vi "WLAN_DPD_AMPM_EVM_SEM.vi"() -> ()   [LabVIEW 2016]
doc: "This example illustrates how to use the RFmx and RFSG drivers and the WLAN toolkit to perform SEM and EVM measurements with or without digital predistortion (DPD) of the waveform input to the DUT. \n\nDPD is a technique to optimize the operating point of power amplifiers and other non-linear RFIC devices. Power amplifiers are much more efficient if they operate near compression. However, compressing signal amplitudes can significantly deteriorate the amplified signal's quality both, in-band (e.g., EVM increases due to non-linear distortion of the signal's I/Q constellation) and out-of-band (e.g., SEM test fails due to spectral regrowth). With DPD, the original waveform is first pre-distorted in a way that matches the non-linear effects of the RFIC device before being fed through the device. The resulting output is a much cleaner amplified and/or filtered version of the original waveform. \n\nDifferent DPD models can be used to trade off performance with computational ease, with the Lookup-Table (LUT) model the simplest and the Generalized Memory Polynomial Model (GMP) the most complex. With a LUT, the DPD algorithm achieves gain and phase linearization on average. If you want to correct for memory effects - i.e., an output sample not only depends on the current input but also previous input samples; you will notice that a specific input power value translates into a range of gain and phase values - you would use one of the memory polynomial models. For these models, several parameters such as polynomial order and memory depth are available to fine-tune the model to the DUT behavior."
uses:
  Source/SG/Typedefs/Instrument Configuration.ctl
  <instrlib>/niRFSG/niRFSG.llb/niRFSG Ref Clock Sources.ctl
  Source/Common/Local Oscillator Sharing Mode.ctl
  <instrlib>/niRFSG/niRFSG.llb/niRFSG Exported Signal Destinations.ctl
  Source/SA/RFmxSpecAn/Typedefs/SpecAn AMPM Results.ctl
  Source/SA/RFmxWLAN/Typedefs/WLAN OFDM ModAcc Configuration.ctl
  Source/Common/SA Common Configuration.ctl
  Source/SA/RFmxWLAN/Typedefs/WLAN Standard Configuration.ctl
  Source/SA/RFmxWLAN/Typedefs/WLAN OFDM ModAcc Results.ctl
  Source/SA/RFmxSpecAn/Typedefs/SpecAn AMPM Configuration.ctl
  Source/Common/Waveform.ctl
  Source/SA/RFmxWLAN/Typedefs/WLAN SEM Configuration.ctl
  Source/SA/RFmxWLAN/Typedefs/WLAN SEM Results.ctl
  Source/Methods/RFmxDPD/Typedefs/Common Configuration.ctl
  Source/Methods/RFmxDPD/Typedefs/Memory Polynomial Configuration.ctl
  Source/SA/RFmxInstr/Typedefs/Instrument Configuration.ctl
  Source/Methods/RFmxDPD/Typedefs/Apply DPD Crest Factor Reduction Configuration.ctl
  Source/Methods/RFmxDPD/Typedefs/Pre DPD Crest Factor Reduction Configuration.ctl
  Source/Methods/RFmxDPD/Typedefs/Pre DPD Crest Factor Reduction Carrier Channel.ctl
  Source/Common/SA Auto Level Configuration.ctl
  <vilib>/RFmx/SpecAn/mx/RFmxSpecAn.llb/RFmxSpecAn AMPM Fetch AM to AM Trace.vi
  <vilib>/RFmx/SpecAn/mx/RFmxSpecAn.llb/RFmxSpecAn AMPM Fetch AM to PM Trace.vi
  <vilib>/RFmx/WLAN/mx/RFmxWLAN.llb/RFmxWLAN OFDMModAcc Fetch Data Constellation Trace.vi
  <vilib>/RFmx/WLAN/mx/RFmxWLAN.llb/RFmxWLAN OFDMModAcc Fetch Pilot Constellation Trace.vi
  <vilib>/RFmx/WLAN/mx/RFmxWLAN.llb/RFmxWLAN SEM Fetch Spectrum.vi
  Source/SG/SG.lvlib
  Source/SA/RFmxWLAN/RFmxWLAN.lvlib
  Source/SA/RFmxSpecAn/RFmxSpecAn.lvlib
  Source/Methods/RFmxDPD/RFmxDPD.lvlib
  Source/Common/Common.lvlib
  Source/SA/RFmxInstr/RFmxInstr.lvlib
panel:
  in  "Error Tab Control":enum32{"Page 1", "Page 2"}(tab)
  out "error out":errorcluster
  in  "Display Tab Control":T1(tab)
  out "AMPM Measurement Results":T2 {"AM to PM Residual (deg)" format="%.2f"; "AM to AM Residual (dB)" format="%.2f"; "Mean RMS EVM (%)" format="%.2f"; "1 dB Compression Point (dBm)" format="%.2f"; "Mean Linear Gain (dB)" format="%.2f"}
  out "AM to PM Plot":T3(graph)
  out "AM to AM Plot":T4(graph)
  out "Constellation":cluster{sgl[], sgl[]}[](graph)
  out "OFDM ModAcc Results":T5 {"Composite Pilot RMS EVM Mean (dB)" format="%.2f"; "Composite Data RMS EVM Mean (dB)" format="%.2f"; "Composite RMS EVM Mean (dB)" format="%.2f"}
  out "SEM Mask":cluster{"x0":dbl, "dx":dbl, "y":sgl[]}[](graph)
  out "WLAN SEM Results":T6 {"Upper Offset Margin Relative Power (dB)" format="%.2f"; "Upper Offset Margin Absolute Power (dBm)" format="%.2f"; "Upper Offset Margin Frequency (Hz)" format="%.3p"; "Upper Offset Margin (dB)" format="%.2f"; "Upper Offset Measurement Status" items=["Fail", "Pass"]; "Lower Offset Margin Relative Power (dB)" format="%.2f"; "Lower Offset Margin Absolute Power (dBm)" format="%.2f"; "Lower Offset Margin Frequency (Hz)" format="%.3p"; "Lower Offset Margin (dB)" format="%.2f"; "Lower Offset Measurement Status" items=["Fail", "Pass"]; "Relative Power (dB)" format="%.2f"; "Absolute Power (dBm)" format="%.2f"; "Measurement Status" items=["Fail", "Pass"]}
  out "Reference Waveform":cluster{"t0":dbl, "dt":dbl, "y":sgl[]}(graph)
  in  "Measurement Settings Tab Control":T7(tab)
  in  "RFmx SpecAn AMPM Configuration":T8={"Measurement Interval (s)"=0.0001, "DUT Average Input Power (dBm)"=-20.0, "Signal Type"=0, "Averaging Enabled"=0, "Averaging Count"=10, "Reference Waveform"={"Name"="Wfm", "Data"=refnum, "Signal Bandwidth (Hz)"=0.0, "PAPR (dB)"=0.0, "Burst Length (s)"=0.0, "Sample Rate"=0.0, "Burst Start Locations"=[], "Burst Stop Locations"=[], "Idle Duration Present?"=FALSE, "Runtime Scaling"=0.0, "Script"=""}} {"Reference Waveform"."Runtime Scaling" format="%#_6p"; "Reference Waveform"."Sample Rate" format="%#_6p"; "Reference Waveform"."Burst Length (s)" format="%#_6p"; "Reference Waveform"."PAPR (dB)" format="%.2f"; "Reference Waveform"."Signal Bandwidth (Hz)" format="%#_6p"; "Averaging Enabled" items=["False", "True"]; "Signal Type" items=["Modulated", "Tones"]; "DUT Average Input Power (dBm)" format="%.2f"; "Measurement Interval (s)" format="%.2p"}
  in  "Common DPD Configuration":T10={"Measurement Interval (s)"=0.0001, "Signal Type"=0, "DUT Average Input Power (dBm)"=-15.0, "Synchronization Method"=1} {"Synchronization Method" items=["Direct"=1, "Alias Protected"=2]; "DUT Average Input Power (dBm)" format="%.2f"; "Signal Type" items=["Modulated", "Tones"]; "Measurement Interval (s)" format="%#.2p"}
  in  "Memory Polynomial Configuration":T11={"Correction Type"=0, "Number of Iterations"=1, " Order"=3, " Depth"=2, "Lead Order"=2, "Lag Order"=2, "Lead Memory Depth"=2, "Lag Memory Depth"=2, "Maximum Lead"=2, "Maximum Lag"=2} {"Order" min=1; "Correction Type" items=["Magnitude and Phase", "Magnitude Only", "Phase Only"]}
  in  "Enable DPD":bool=TRUE
  in  "Pre DPD Crest Factor Reduction":T12={"Enabled"=0, "Method"=0, "Max Iterations"=10, "Target PAPR (dB)"=8.0, "Shaping Factor"=5.0, "Shaping Threshold (dB)"=-5.0, "Window Type"=7, "Window Length"=10, "Filter Enabled"=0, "Carrier Channels"=[{"Offset (Hz)"=0.0, "Bandwidth (Hz)"=20000000.0}]} {"Carrier Channels"."Bandwidth (Hz)" format="%.2p"; "Carrier Channels"."Offset (Hz)" format="%.2p"; "Filter Enabled" items=["False", "True"]; "Window Type" items=["Flat Top"=1, "Hanning"=2, "Hamming"=3, "Gaussian"=4, "Blackman"=5, "Blackman-Harris"=6, "Kaiser-Bessel"=7]; "Method" items=["Clipping", "Peak Windowing", "Sigmoid"]; "Enabled" items=["False", "True"]}
  in  "Apply DPD Crest Factor Reduction":T14={"Enabled"=0, "Method"=0, "Max Iterations"=10, "Target PAPR Type"=0, "Target PAPR (dB)"=8.0, "Window Type"=7, "Window Length"=10, "Shaping Factor"=5.0, "Shaping Threshold (dB)"=-5.0} {"Target PAPR Type" items=["Input PAPR", "Custom"]; "Window Type" items=["Flat Top"=1, "Hanning"=2, "Hamming"=3, "Gaussian"=4, "Blackman"=5, "Blackman-Harris"=6, "Kaiser-Bessel"=7]; "Method" items=["Clipping", "Peak Windowing", "Sigmoid"]; "Enabled" items=["False", "True"]}
  in  "OFDM ModAcc Configuration":T15={"Acquisition Length (s)"=0.0, "Averaging Enabled"=0, "Averaging Count"=10, "Optimize Dynamic Range for EVM Enabled"=1, "Optimize Dynamic Range for EVM Margin (dB)"=0.0, "Measurement Offset (sym)"=0, "Maximum Measurement Length (sym)"=16} {"Optimize Dynamic Range for EVM Margin (dB)" format="%.2f"; "Optimize Dynamic Range for EVM Enabled" items=["False", "True"]; "Averaging Enabled" items=["False", "True"]; "Acquisition Length (s)" format="%.3p"}
  in  "WLAN SEM Configuration":T16={"Sweep Time Auto"=1, "Sweep Time (s)"=0.001, "Span Auto"=1, "Span (Hz)"=100000000.0, "Averaging Enabled"=0, "Averaging Count"=5, "Averaging Type"=0} {"Averaging Type" items=["RMS", "Log", "Scalar", "Max", "Min"]; "Averaging Enabled" items=["False", "True"]; "Span (Hz)" format="%.3p"; "Span Auto" items=["False", "True"]; "Sweep Time (s)" format="%.3p"; "Sweep Time Auto" items=["False", "True"]}
  in  "Center Frequency (Hz)":dbl=5180000000.0 format="%.6p"
  out "Resource Control":enum32{"RFSG", "RFSA", "WLAN Signal"}(tab)
  in  "Reference Waveform File Path":path=path "C:/Users/Public/Documents/National Instruments/RFIC Test Software/Waveforms/80211ax_80M_MCS11.tdms"
  in  "RFSG Resource Name":refnum<k15>="5840"
  in  "SG Configuration":T17={"SelectedPorts"="", "Reference Clock Source"="PXI_CLK", "Carrier Frequency (Hz)"=1000000000.0, "DUT Average Input Power (dBm)"=-10.0, "External Attenuation (dB)"=0.0, "LO Sharing Mode"=enum."Automatic"}
  in  "Marker Event Output Terminal":T20="PXI_Trig0"
  in  "RFSA Resource Name":refnum<k15>="5840" caption="Resource Name"
  in  "Common Configuration":T21={"Center Frequency (Hz)"=1000000000.0, "Reference Level (dBm)"=0.0, "External Attenuation (dB)"=0.0, "Trigger Enabled"=TRUE, "Digital Trigger Source"="PXI_Trig0", "Trigger Delay (s)"=0.0, "Selected Ports"=""} {"Trigger Delay (s)" format="%.2p"; "External Attenuation (dB)" format="%.2f"; "Reference Level (dBm)" format="%.2f"; "Center Frequency (Hz)" format="%.6p"}
  in  "Instrument Configuration":T22={"LO Sharing Mode"=enum."Automatic", "Frequency Reference Source"="PXI_Clk"}
  in  "Auto Level Configuration":T23={"Enabled"=FALSE, "Measurement Interval (s)"=0.01} {"Measurement Interval (s)" min=1e-06 max=100.0 format="%.2p"}
  in  "WLAN Signal Configuration":T24={"Standard"=6, "Channel Bandwidth (Hz)"=80000000.0} {"Channel Bandwidth (Hz)" items=["5M"=5000000.0, "10M"=10000000.0, "20M"=20000000.0, "40M"=40000000.0, "80M"=80000000.0, "160M"=160000000.0]; "Standard" items=["802.11a/g", "802.11b", "802.11j", "802.11p", "802.11n", "802.11ac", "802.11ax"]}
  # "This example supports waveforms generated by the NI WLAN Generation Toolkit/Soft Front Panel and stored in the TDMS file format. Preferably, the waveform starts with one WLAN burst followed by idle time. The waveform headroom should account for the PAPR plus some margin (say 1.5 dB)."
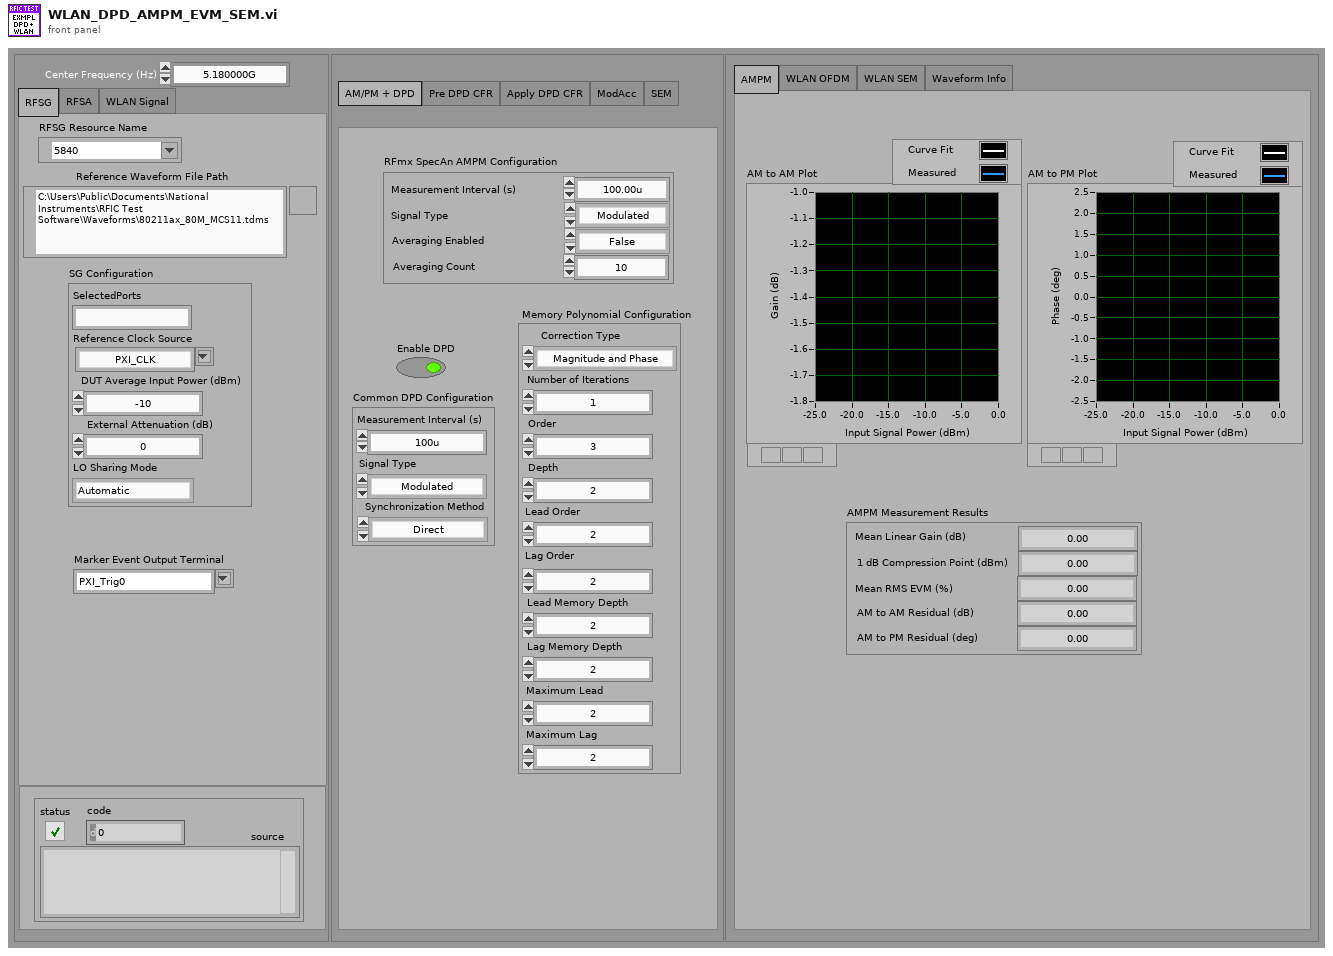
[diagram p1: front panel]
types:
  T1 = enum32{"AMPM", "WLAN OFDM", "WLAN SEM", "Waveform Info"}
  T2 = typedef "RFmxSpecAn.lvlib/SpecAn AMPM Results.ctl" = cluster{"Mean Linear Gain (dB)":dbl, "1 dB Compression Point (dBm)":dbl, "Mean RMS EVM (%)":dbl, "AM to AM Residual (dB)":dbl, "AM to PM Residual (deg)":dbl}
  T3 = cluster{"Input Powers (dBm)":sgl[], "Curve Fit AM to PM (dB)":sgl[]}[]
  T4 = cluster{"Input Powers (dBm)":sgl[], "Curve Fit AM to AM (dB)":sgl[]}[]
  T5 = typedef "RFmxWLAN.lvlib/WLAN OFDM ModAcc Results.ctl" = cluster{"Composite RMS EVM Mean (dB)":dbl, "Composite Data RMS EVM Mean (dB)":dbl, "Composite Pilot RMS EVM Mean (dB)":dbl, "Number of Symbols Used":i32}
  T6 = typedef "RFmxWLAN.lvlib/WLAN SEM Results.ctl" = cluster{"Measurement Status":i32, "Absolute Power (dBm)":dbl, "Relative Power (dB)":dbl, "Lower Offset Measurement Status":i32[], "Lower Offset Margin (dB)":dbl[], "Lower Offset Margin Frequency (Hz)":dbl[], "Lower Offset Margin Absolute Power (dBm)":dbl[], "Lower Offset Margin Relative Power (dB)":dbl[], "Upper Offset Measurement Status":i32[], "Upper Offset Margin (dB)":dbl[], "Upper Offset Margin Frequency (Hz)":dbl[], "Upper Offset Margin Absolute Power (dBm)":dbl[], "Upper Offset Margin Relative Power (dB)":dbl[]}
  T7 = enum32{"AM/PM + DPD", "Pre DPD CFR", "Apply DPD CFR", "ModAcc", "SEM"}
  T8 = typedef "RFmxSpecAn.lvlib/SpecAn AMPM Configuration.ctl" = cluster{"Measurement Interval (s)":dbl, "DUT Average Input Power (dBm)":dbl, "Signal Type":i32, "Averaging Enabled":i32, "Averaging Count":i32, "Reference Waveform":T9}
  T9 = typedef "Common.lvlib/Waveform.ctl" = cluster{"Name":string, "Data":refnum<data-value>, "Signal Bandwidth (Hz)":dbl, "PAPR (dB)":dbl, "Burst Length (s)":dbl, "Sample Rate":dbl, "Burst Start Locations":i32[], "Burst Stop Locations":i32[], "Idle Duration Present?":bool, "Runtime Scaling":dbl, "Script":string}
  T10 = typedef "RFmxDPD.lvlib/Common Configuration.ctl" = cluster{"Measurement Interval (s)":dbl, "Signal Type":i32, "DUT Average Input Power (dBm)":dbl, "Synchronization Method":i32}
  T11 = typedef "RFmxDPD.lvlib/Memory Polynomial Configuration.ctl" = cluster{"Correction Type":i32, "Number of Iterations":i32, " Order":i32, " Depth":i32, "Lead Order":i32, "Lag Order":i32, "Lead Memory Depth":i32, "Lag Memory Depth":i32, "Maximum Lead":i32, "Maximum Lag":i32}
  T12 = typedef "RFmxDPD.lvlib/Pre DPD Crest Factor Reduction Configuration.ctl" = cluster{"Enabled":i32, "Method":i32, "Max Iterations":i32, "Target PAPR (dB)":dbl, "Shaping Factor":dbl, "Shaping Threshold (dB)":dbl, "Window Type":i32, "Window Length":i32, "Filter Enabled":i32, "Carrier Channels":T13[]}
  T13 = typedef "RFmxDPD.lvlib/Pre DPD Crest Factor Reduction Carrier Channel.ctl" = cluster{"Offset (Hz)":dbl, "Bandwidth (Hz)":dbl}
  T14 = typedef "RFmxDPD.lvlib/Apply DPD Crest Factor Reduction Configuration.ctl" = cluster{"Enabled":i32, "Method":i32, "Max Iterations":i32, "Target PAPR Type":i32, "Target PAPR (dB)":dbl, "Window Type":i32, "Window Length":i32, "Shaping Factor":dbl, "Shaping Threshold (dB)":dbl}
  T15 = typedef "RFmxWLAN.lvlib/WLAN OFDM ModAcc Configuration.ctl" = cluster{"Acquisition Length (s)":dbl, "Averaging Enabled":i32, "Averaging Count":i32, "Optimize Dynamic Range for EVM Enabled":i32, "Optimize Dynamic Range for EVM Margin (dB)":dbl, "Measurement Offset (sym)":i32, "Maximum Measurement Length (sym)":i32}
  T16 = typedef "RFmxWLAN.lvlib/WLAN SEM Configuration.ctl" = cluster{"Sweep Time Auto":i32, "Sweep Time (s)":dbl, "Span Auto":i32, "Span (Hz)":dbl, "Averaging Enabled":i32, "Averaging Count":i32, "Averaging Type":i32}
  T17 = typedef "SG.lvlib/Instrument Configuration.ctl" = cluster{"SelectedPorts":string, "Reference Clock Source":T18, "Carrier Frequency (Hz)":dbl, "DUT Average Input Power (dBm)":dbl, "External Attenuation (dB)":dbl, "LO Sharing Mode":T19}
  T18 = typedef "niRFSG Ref Clock Sources.ctl" = string
  T19 = typedef "Common.lvlib/Local Oscillator Sharing Mode.ctl" = enum16{"Automatic", "None"}
  T20 = typedef "niRFSG Exported Signal Destinations.ctl" = string
  T21 = typedef "Common.lvlib/SA Common Configuration.ctl" = cluster{"Center Frequency (Hz)":dbl, "Reference Level (dBm)":dbl, "External Attenuation (dB)":dbl, "Trigger Enabled":bool, "Digital Trigger Source":string, "Trigger Delay (s)":dbl, "Selected Ports":string}
  T22 = typedef "RFmxInstr.lvlib/Instrument Configuration.ctl" = cluster{"LO Sharing Mode":T19, "Frequency Reference Source":string}
  T23 = typedef "Common.lvlib/SA Auto Level Configuration.ctl" = cluster{"Enabled":bool, "Measurement Interval (s)":dbl}
  T24 = typedef "RFmxWLAN.lvlib/WLAN Standard Configuration.ctl" = cluster{"Standard":i32, "Channel Bandwidth (Hz)":dbl}
  T25 = enum16{"TXP", "PowerRamp", "DSSSModAcc", "OFDMModAcc", "SEM"}[]
  T26 = enum16{"ACP", "CCDF", "CHP", "FCnt", "Harmonics", "OBW", "SEM", "Spectrum", "Spur", "TXP", "AMPM", "DPD", "IQ", "IM", "NF", "PhaseNoise", "PAVT"}[]
  T27 = cluster{"Reference Powers (dBm)":sgl[], "Curve Fit AM to AM (dB)":sgl[]}
  T28 = cluster{"Reference Powers (dBm)":sgl[], "Measured AM to AM (dB)":sgl[]}
  T29 = cluster{"Reference Powers (dBm)":sgl[], "Curve Fit AM to PM (deg)":sgl[]}
  T30 = cluster{"Reference Powers (dBm)":sgl[], "Measured AM to PM (deg)":sgl[]}
  T31 = cluster{"Reference Powers (dBm)":sgl[], "Measured AM to AM (dB)":sgl[]}[]
  T32 = cluster{"Reference Powers (dBm)":sgl[], "Measured AM to PM (deg)":sgl[]}[]
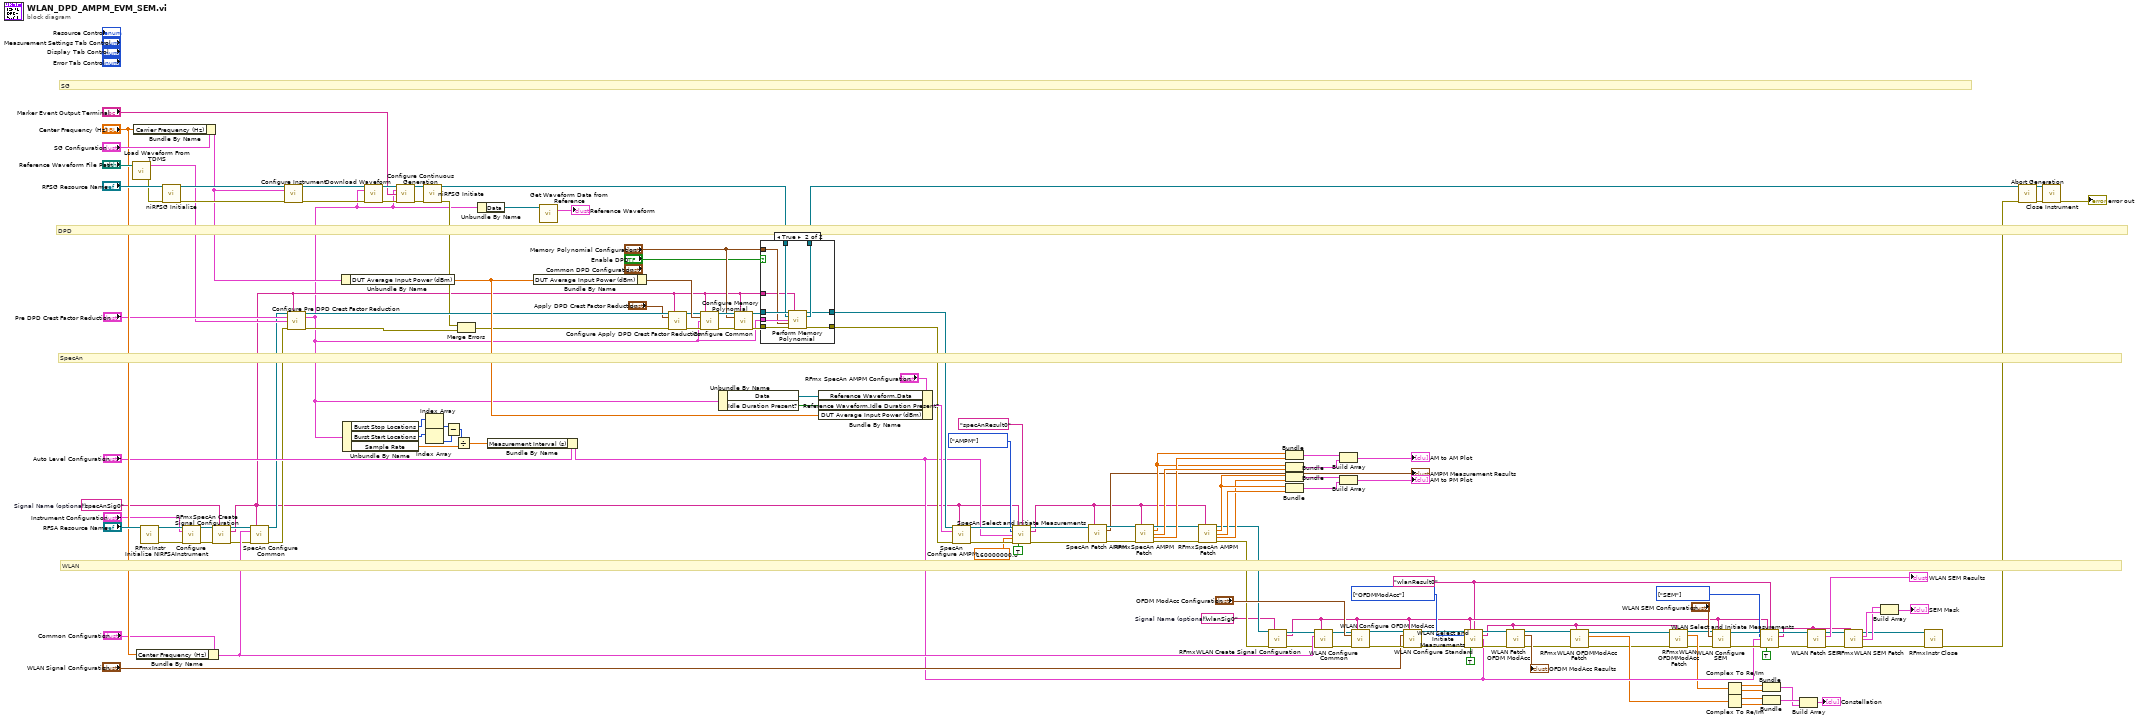
[diagram p0: block diagram]
diagram:
  w5 = "wlanResult0" ("Result Name")
  w14 = "specAnSig0"  # Signal Name (optional)
  w10 = "wlanSig0"  # Signal Name (optional)
  w41 = T25 [enum."SEM"] items=["TXP", "PowerRamp", "DSSSModAcc", "OFDMModAcc", "SEM"] ("Measurements")
  w49 = T25 [enum."OFDMModAcc"] items=["TXP", "PowerRamp", "DSSSModAcc", "OFDMModAcc", "SEM"] ("Measurements")
  w55 = T26 [enum."AMPM"] items=["ACP", "CCDF", "CHP", "FCnt", "Harmonics", "OBW", "SEM", "Spectrum", "Spur", "TXP", "AMPM", "DPD", "IQ", "IM", "NF", "PhaseNoise", "PAVT"] ("Measurements")
  # "SpecAn"
  # "WLAN"
  # "DPD"
  # "SG"
  n1 = call "Load Waveform From TDMS.vi"("TDMS File Path"="Reference Waveform File Path") -> ("Waveform"=w23:T9, "error out"=w127:errorcluster)  [unwired: 13 in]
  n2 = Bundle By Name(cluster="SG Configuration", "Carrier Frequency (Hz)"="Center Frequency (Hz)") -> (w83:T17)
  n3 = Bundle By Name(cluster="Common Configuration", "Center Frequency (Hz)"="Center Frequency (Hz)") -> (w72:T21)
  n4 = call <vilib>:"RFmxInstr Initialize NIRFSA.vi"("Resource Name"="RFSA Resource Name") -> ("Instrument Handle Out"=w70:refnum<k21>, "error out"=w69:errorcluster)  [unwired: 12 in, 1 out]
  n5 = call <instrlib>:"niRFSG Initialize.vi"("resource name"="RFSG Resource Name", "error in"=w127) -> ("instrument handle"=w144:refnum<k15>, "error out"=w143:errorcluster)  [unwired: 12 in]
  n6 = call "Configure Instrument.vi"("Instrument Handle In"=w70, "Instrument Configuration"="Instrument Configuration", "error in (no error)"=w69) -> ("Instrument Handle Out"=w22:refnum<k21>, "error out"=w21:errorcluster)  [unwired: 11 in]
  n7 = call <vilib>:"RFmxSpecAn Create Signal Configuration.vi"("Instrument Handle In"=w22, "Signal Name"=w14, "error in (no error)"=w21) -> ("Instrument Handle Out"=w19:refnum<k21>, "Selector String Out"=w4:string, "error out"=w20:errorcluster)  [unwired: 10 in]
  n8 = call "SpecAn Configure Common.vi"("RFmx Handle In"=w19, "Selector String"=w4, "Common Configuration"=w72) -> ("RFmx Handle Out"=w18:refnum<k21>)  [unwired: 11 in, 1 out]
  n9 = call "Configure Instrument.vi"("RFSG Session In"=w144, "SG Configuration"=w83, "error in (no error)"=w143) -> ("RFSG Session Out"=w145:refnum<k15>, "error out"=w126:errorcluster)  [unwired: 11 in]
  n10 = call "Configure Pre DPD Crest Factor Reduction.vi"("Instrument Handle In"=w18, "Selector String"=w4, "Pre DPD Crest Factor Reduction Configuration"="Pre DPD Crest Factor Reduction", "Reference Waveform"=w23, "error in (no error)"=w20) -> ("Instrument Handle Out"=w71:refnum<k21>, "Pre DPD CFR Waveform"=w1:T9, "error out"=w16:errorcluster)  [unwired: 8 in]
  n11 = Unbundle By Name(w83) -> ("DUT Average Input Power (dBm)"=w75:dbl)
  n12 = Unbundle By Name(w1) -> ("Burst Stop Locations"=w125:i32[], "Burst Start Locations"=w124:i32[], "Sample Rate"=w120:dbl)
  n13 = call "Download Waveform.vi"("RFSG handle"=w145, "Waveform In"=w1, "error in (no error)"=w126) -> ("RFSG handle out"=w142:refnum<k15>, "error out"=w141:errorcluster)  [unwired: 11 in]
  n14 = call "Configure Continuous Generation.vi"("RFSG handle"=w142, "Waveform in"=w1, "Waveform Start Trigger Export"="Marker Event Output Terminal", "error in"=w141) -> ("RFSG handle out"=w119:refnum<k15>, "error out"=w118:errorcluster)  [unwired: 9 in, 1 out]
  n15 = call <instrlib>:"niRFSG Initiate.vi"("instrument handle"=w119, "error in"=w118) -> ("instrument handle out"=w87:refnum<k15>, "error out"=w17:errorcluster)  [unwired: 12 in]
  n16 = Index Array(array=w125) -> (element=w123:i32)  [unwired: 1 in]
  n17 = Index Array(array=w124) -> (element=w122:i32)  [unwired: 1 in]
  n18 = Subtract(x=w123, y=w122) -> (x-y=w121:i32)
  n19 = Divide(x=w121, y=w120) -> (x/y=w46:dbl)
  n20 = Merge Errors(w17, w16) -> (w15:errorcluster)
  n21 = Unbundle By Name(w1) -> ("Data"=w74:refnum<data-value>)
  n22 = Bundle By Name(cluster="Auto Level Configuration", "Measurement Interval (s)"=w46) -> (w39:T23)
  n23 = Bundle By Name(cluster="Common DPD Configuration", "DUT Average Input Power (dBm)"=w75) -> (w84:T10)
  n24 = call "Get Waveform Data from Reference.vi"("Waveform Data Reference"=w74) -> ("Waveform Data"=→"Reference Waveform":cluster{"t0":dbl, "dt":dbl, "y":csg[]})  [unwired: 13 in, 1 out]
  n25 = call "Configure Apply DPD Crest Factor Reduction.vi"("Instrument Handle In"=w71, "Selector String"=w4, "Apply DPD Crest Factor Reduction Configuration"="Apply DPD Crest Factor Reduction", "error in (no error)"=w15) -> ("Instrument Handle Out"=w66:refnum<k21>, "error out"=w67:errorcluster)  [unwired: 10 in]
  n26 = call "Configure Common.vi"("Instrument Handle In"=w66, "Selector String"=w4, "Common Configuration"=w84, "Reference Waveform"=w1, "error in (no error)"=w67) -> ("Instrument Handle Out"=w91:refnum<k21>, "error out"=w90:errorcluster)  [unwired: 9 in]
  n27 = Unbundle By Name(w1) -> ("Data"=w132:refnum<data-value>, "Idle Duration Present?"=w116:bool)
  n28 = call "Configure Memory Polynomial.vi"("Instrument Handle In"=w91, "Selector String"=w4, "Memory Polynomial Configuration"="Memory Polynomial Configuration", "error in (no error)"=w90) -> ("Instrument Handle Out"=w89:refnum<k21>, "error out"=w88:errorcluster)  [unwired: 10 in]
  n29 = case shown="True" "Enable DPD" {
    tunnel: w89 -> [w150 w160]
    tunnel: [w149 w159] -> w77
    tunnel: "Memory Polynomial Configuration" -> [_ w153]
    tunnel: w1 -> [_ w158]
    tunnel: w87 -> [w151 w157]
    tunnel: [w151 w156] -> w86
    tunnel: [w150 w155] -> w76
    tunnel: w88 -> [w149 w154]
    tunnel: w4 -> [_ w152]
    frame False {
    }
    frame True {
      n30 = call "Perform Memory Polynomial.vi"("RFmx Instrument Handle In"=w160, "Selector String"=w152, "RFSG Instrument Handle In"=w157, "Reference Waveform"=w158, "Memory Polynomial Configuration"=w153, "error in (no error)"=w154) -> ("RFmx Instrument Handle Out"=w155:refnum<k21>, "RFSG Instrument Handle Out"=w156:refnum<k15>, "error out"=w159:errorcluster)  [unwired: 6 in, 1 out]
    }
  }
  n31 = Bundle By Name(cluster="RFmx SpecAn AMPM Configuration", "Reference Waveform.Data"=w132, "Reference Waveform.Idle Duration Present?"=w116, "DUT Average Input Power (dBm)"=w75) -> (w133:T8)
  n32 = call "SpecAn Configure AMPM.vi"("RFmx Handle In"=w76, "Selector String"=w4, "RFmx SpecAn AMPM Configuration"=w133, "error in (no error)"=w77) -> ("RFmx Handle Out"=w60:refnum<k21>, "error out"=w59:errorcluster)  [unwired: 10 in]
  n33 = call "SpecAn Select and Initiate Measurements.vi"("Instrument Handle In"=w60, "Selector String"=w4, "Result Name"="specAnResult0", "Measurements"=w55, "Auto Level Configuration"=w39, "Auto Level Bandwidth (Hz)"=160000000.0, "error in (no error)"=w59, "Enable All Traces (F)"=TRUE) -> ("Instrument Handle Out"=w58:refnum<k21>, "Selector String Out"=w2:string, "error out"=w57:errorcluster)  [unwired: 5 in]
  n34 = call "SpecAn Fetch AMPM.vi"("RFmx Handle In"=w58, "Selector String"=w2, "error in (no error)"=w57) -> ("RFmx Handle Out"=w104:refnum<k21>, "AMPM Results"=→"AMPM Measurement Results":T2, "error out"=w103:errorcluster)  [unwired: 10 in]
  n35 = call-poly <vilib>:"RFmxSpecAn AMPM Fetch.vi"("Instrument Handle In"=w104, "Selector String"=w2, "error in (no error)"=w103) -> ("Instrument Handle Out"=w110:refnum<k21>, "Reference Powers (dBm)"=w102:sgl[], "Measured AM to AM (dB)"=w115:sgl[], "Curve Fit AM to AM (dB)"=w114:sgl[], "error out"=w109:errorcluster)  [unwired: 8 in]
  n36 = call-poly <vilib>:"RFmxSpecAn AMPM Fetch.vi"("Instrument Handle In"=w110, "Selector String"=w2, "error in (no error)"=w109) -> ("Instrument Handle Out"=w13:refnum<k21>, "Reference Powers (dBm)"=w113:sgl[], "Measured AM to PM (deg)"=w112:sgl[], "Curve Fit AM to PM (deg)"=w111:sgl[], "error out"=w12:errorcluster)  [unwired: 8 in]
  n37 = call <vilib>:"RFmxWLAN Create Signal Configuration.vi"("Instrument Handle In"=w13, "Signal Name"=w10, "error in (no error)"=w12) -> ("Instrument Handle Out"=w11:refnum<k21>, "Selector String Out"=w7:string, "error out"=w9:errorcluster)  [unwired: 10 in]
  n38 = Bundle("Reference Powers (dBm)"=w102, "Curve Fit AM to AM (dB)"=w114) -> (w108:T27)  [unwired: 1 in]
  n39 = Bundle("Reference Powers (dBm)"=w102, "Measured AM to AM (dB)"=w115) -> (w107:T28)  [unwired: 1 in]
  n40 = Bundle("Reference Powers (dBm)"=w113, "Curve Fit AM to PM (deg)"=w111) -> (w105:T29)  [unwired: 1 in]
  n41 = Bundle("Reference Powers (dBm)"=w113, "Measured AM to PM (deg)"=w112) -> (w106:T30)  [unwired: 1 in]
  n42 = call "WLAN Configure Common.vi"("Instrument Handle In"=w11, "Selector String"=w7, "Common Configuration"=w72, "error in (no error)"=w9) -> ("Instrument Handle Out"=w80:refnum<k21>, "error out"=w79:errorcluster)  [unwired: 10 in]
  n43 = Build Array(w108, w107) -> (→"AM to AM Plot":T31)
  n44 = Build Array(w105, w106) -> (→"AM to PM Plot":T32)
  n45 = call "WLAN Configure OFDM ModAcc.vi"("Instrument Handle In"=w80, "Selector String"=w7, "OFDM ModAcc Configuration"="OFDM ModAcc Configuration", "error in (no error)"=w79) -> ("Instrument Handle Out"=w78:refnum<k21>, "error out"=w134:errorcluster)  [unwired: 10 in]
  n46 = call "WLAN Configure Standard.vi"("Instrument Handle In"=w78, "Selector String"=w7, "WLAN Standard Configuration"="WLAN Signal Configuration", "error in (no error)"=w134) -> ("Instrument Handle Out"=w53:refnum<k21>, "error out"=w52:errorcluster)  [unwired: 10 in]
  n47 = call "WLAN Select and Initiate Measurements.vi"("Instrument Handle In"=w53, "Selector String"=w7, "Result Name"=w5, "Measurements"=w49, "Auto Level Configuration"=w39, "error in (no error)"=w52, "Enable All Traces (F)"=TRUE) -> ("Instrument Handle Out"=w51:refnum<k21>, "Selector String Out"=w8:string, "error out"=w50:errorcluster)  [unwired: 6 in]
  n48 = call "WLAN Fetch OFDM ModAcc.vi"("Instrument Handle In"=w51, "Selector String"=w8, "error in (no error)"=w50) -> ("Instrument Handle Out"=w28:refnum<k21>, "OFDM ModAcc Results"=→"OFDM ModAcc Results":T5, "error out"=w27:errorcluster)  [unwired: 10 in]
  n49 = call-poly <vilib>:"RFmxWLAN OFDMModAcc Fetch.vi"("Instrument Handle In"=w28, "Selector String"=w8, "error in (no error)"=w27) -> ("Instrument Handle Out"=w38:refnum<k21>, "Data Constellation"=w36:csg[], "error out"=w29:errorcluster)  [unwired: 10 in]
  n50 = call-poly <vilib>:"RFmxWLAN OFDMModAcc Fetch.vi"("Instrument Handle In"=w38, "Selector String"=w8, "error in (no error)"=w29) -> ("Instrument Handle Out"=w26:refnum<k21>, "Pilot Constellation"=w37:csg[], "error out"=w25:errorcluster)  [unwired: 10 in]
  n51 = call "WLAN Configure SEM.vi"("Instrument Handle In"=w26, "Selector String"=w7, "WLAN SEM Configuration"="WLAN SEM Configuration", "error in (no error)"=w25) -> ("Instrument Handle Out"=w45:refnum<k21>, "error out"=w43:errorcluster)  [unwired: 10 in]
  n52 = Complex To Re/Im(x + iy=w37) -> (x=w33:sgl[], y=w32:sgl[])
  n53 = Complex To Re/Im(x + iy=w36) -> (x=w35:sgl[], y=w34:sgl[])
  n54 = call "WLAN Select and Initiate Measurements.vi"("Instrument Handle In"=w45, "Selector String"=w7, "Result Name"=w5, "Measurements"=w41, "Auto Level Configuration"=w39, "error in (no error)"=w43, "Enable All Traces (F)"=TRUE) -> ("Instrument Handle Out"=w44:refnum<k21>, "Selector String Out"=w6:string, "error out"=w42:errorcluster)  [unwired: 6 in]
  n55 = Bundle(w35, w34) -> (w31:cluster{sgl[], sgl[]})  [unwired: 1 in]
  n56 = Bundle(w33, w32) -> (w30:cluster{sgl[], sgl[]})  [unwired: 1 in]
  n57 = Build Array(w31, w30) -> (→"Constellation":cluster{sgl[], sgl[]}[])
  n58 = call "WLAN Fetch SEM.vi"("Instrument Handle In"=w44, "Selector String"=w6, "error in (no error)"=w42) -> ("Instrument Handle Out"=w96:refnum<k21>, "WLAN SEM Results"=→"WLAN SEM Results":T6, "error out"=w95:errorcluster)  [unwired: 10 in]
  n59 = call-poly <vilib>:"RFmxWLAN SEM Fetch.vi"("Instrument Handle In"=w96, "Selector String"=w6, "error in (no error)"=w95) -> ("Instrument Handle Out"=w63:refnum<k21>, "Spectrum (dBm)"=w94:cluster{"x0":dbl, "dx":dbl, "y":sgl[]}, "Composite Mask (dBm)"=w93:cluster{"x0":dbl, "dx":dbl, "y":sgl[]}, "error out"=w62:errorcluster)  [unwired: 9 in]
  n60 = Build Array(w93, w94) -> (→"SEM Mask":cluster{"x0":dbl, "dx":dbl, "y":sgl[]}[])
  n61 = call <vilib>:"RFmxInstr Close.vi"("Instrument Handle In"=w63, "error in (no error)"=w62) -> ("error out"=w61:errorcluster)  [unwired: 13 in]
  n62 = call "Abort Generation.vi"("RFSG handle"=w86, "error in (no error)"=w61) -> ("RFSG handle out"=w146:refnum<k15>, "error out"=w147:errorcluster)  [unwired: 12 in]
  n63 = call "Close Instrument.vi"("RFSG Handle"=w146, "error in (no error)"=w147) -> ("error out"=→"error out":errorcluster)  [unwired: 13 in]
